vi "meTEC_Set_ID 3000_Object Target Temperature.vi"(6 "Instance (1)":u8=1, 8 "error in (no error)":errorcluster, 9 "TEC Configuration_IN":T1={"VISA resource name"="", "Device Address"=2}, 10 "Sequence No.":u16=5552, 11 "Object Target Temperature [°C]":dbl=21.75) -> (0 "error out":errorcluster, 1 "TEC Configuration_OUT":T1={"VISA resource name"="", "Device Address"=2}, 3 "Serial Message_Read":string)   [LabVIEW 2019]
uses:
  TypeDefs/meTEC_Configuration.ctl
panel:
  # "--- Inputs ---"
  # "--- Outputs ---"
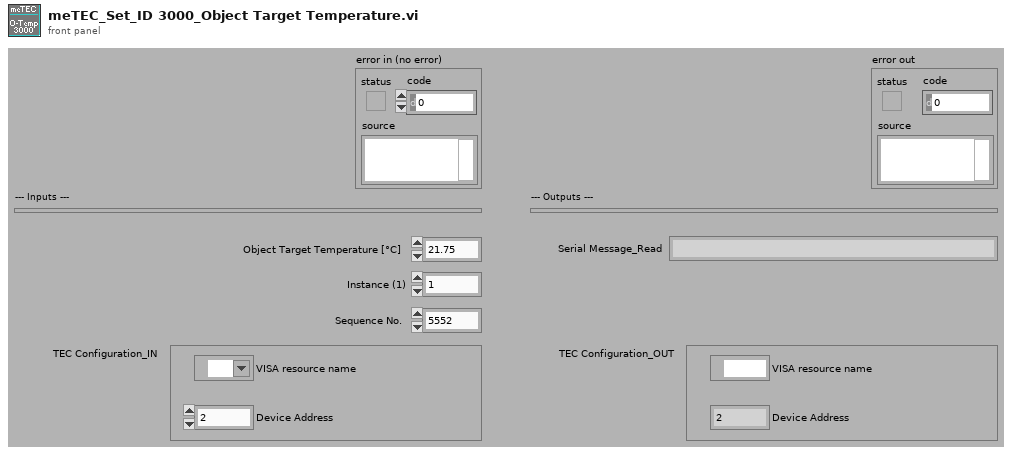
[diagram p1: front panel]
types:
  T1 = typedef "meTEC_Configuration.ctl" = cluster{"VISA resource name":refnum<visa-resource-name>, "Device Address":u16}
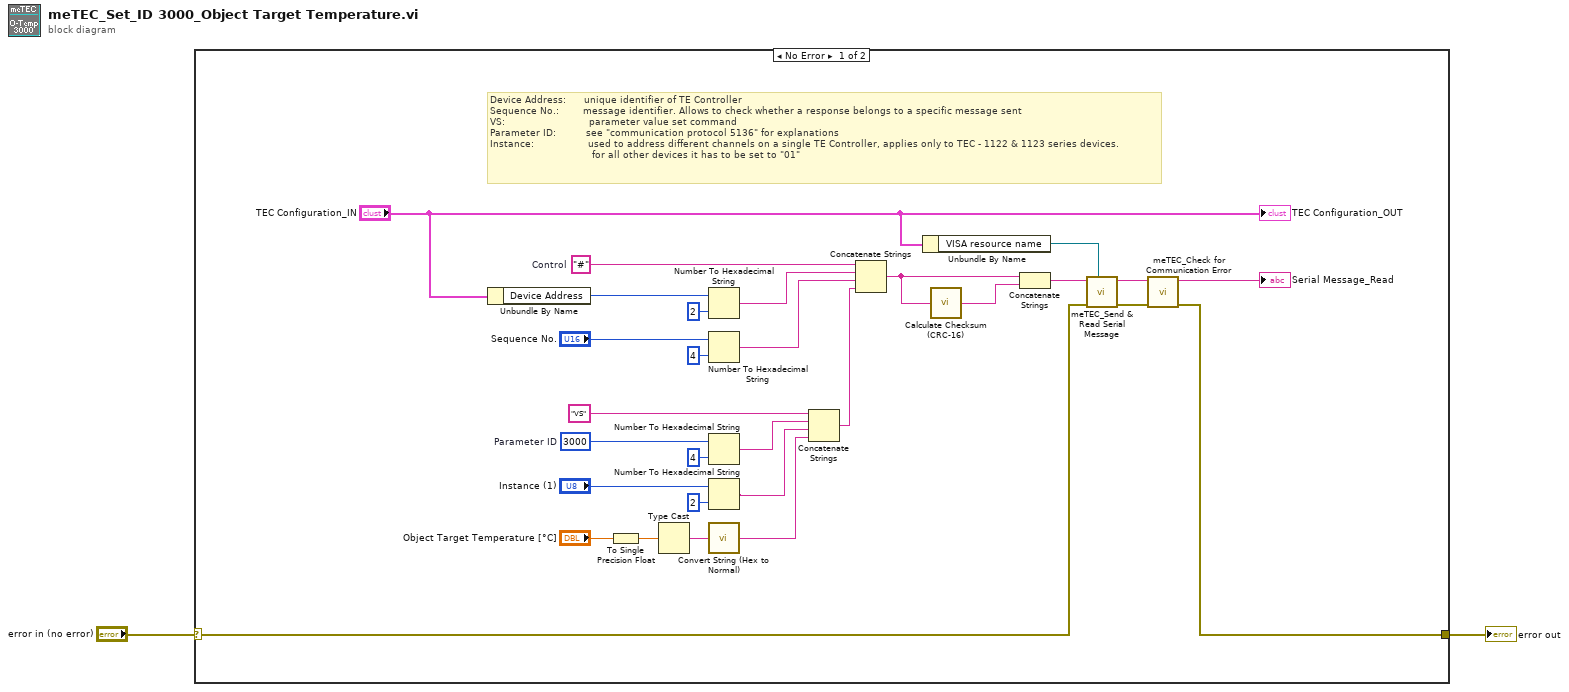
[diagram p0: block diagram]
diagram:
  n1 = case shown="No Error" "error in (no error)" {
    selector: "error in (no error)" -> [w13 w32]
    tunnel: [w5 w32] -> w2
    frame No Error {
      w21 = "#"  # Control
      w30 = 3000  # Parameter ID
      # "Device Address:      unique identifier of TE Controller\nSequence No.:        message identifier. Allows to check whether a response belongs to a specific message sent \nVS:                            parameter value set command\nParameter ID:          see \"communication protocol 5136\" for explanations\nInstance:                  used to address different channels on a single TE Controller, applies only to TEC - 1122 & 1123 series devices.\n                                  for all other devices it has to be set to \"01\""
      n2 = Unbundle By Name("TEC Configuration_IN") -> ("Device Address"=w8:u16)
      n3 = To Single Precision Float(number="Object Target Temperature [°C]") -> (single precision float=w25:sgl)
      n4 = Type Cast(x=w25) -> (*(type *) &x=w24:string)  [unwired: 1 in]
      n5 = Number To Hexadecimal String(1:i16 2 ("width (-)"), 2:w8) -> (0:w16:string)
      n6 = Number To Hexadecimal String(1:i16 4 ("width (-)"), 2:"Sequence No.") -> (0:w20:string)
      n7 = Number To Hexadecimal String(1:i16 4 ("width (-)"), 2:w30) -> (0:w28:string)
      n8 = Number To Hexadecimal String(1:i16 2 ("width (-)"), 2:"Instance (1)") -> (0:w9:string)
      n9 = call "Convert String (Hex to Normal).vi"("Hex String"=w24) -> ("Normal String"=w26:string)  [unwired: 1 in]
      n10 = Concatenate Strings("VS", w28, w9, w26) -> (w15:string)
      n11 = Concatenate Strings(w21, w16, w20, w15) -> (w19:string)
      n12 = Unbundle By Name("TEC Configuration_IN") -> ("VISA resource name"=w11:refnum<visa-resource-name>)
      n13 = call "Calculate Checksum (CRC-16).vi"("Message"=w19) -> ("CRC [String]"=w18:string)  [unwired: 1 in]
      n14 = Concatenate Strings(w19, w18) -> (w14:string)
      n15 = call "meTEC_Send & Read Serial Message.vi"("VISA resource name"=w11, "error in (no error)"=w13, "Serial Message"=w14) -> ("error out"=w12:errorcluster, "Serial Message_Read"=w4:string)  [unwired: 7 in]
      n16 = call "meTEC_Check for Communication Error.vi"("error in (no error)"=w12, "Serial Message_IN"=w4) -> ("error out"=w5:errorcluster, "Serial Message_OUT"=→"Serial Message_Read":string)  [unwired: 8 in]
      "TEC Configuration_OUT" <- "TEC Configuration_IN"
    }
    frame Error {
    }
  }
  "error out" <- w2
